vi "lifetime_error_buffer.vi"(1 "error in":errorcluster, 2 "command":string) -> (0 "error out":errorcluster)   [LabVIEW 2015]
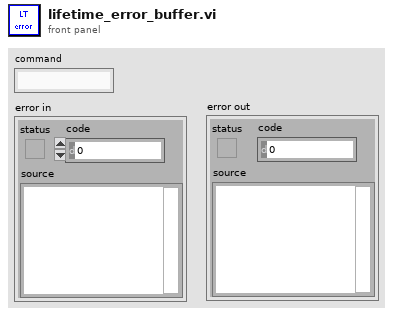
[diagram p1: front panel]
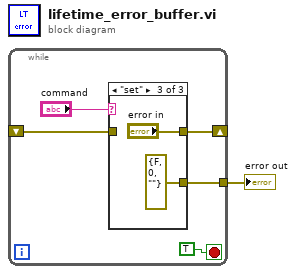
[diagram p0: block diagram]
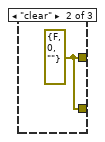
[diagram p3: hidden frame]
diagram:
  n1 = while {
    shift-right: [w4] -> _
    shift-left: _ -> [w3]
    tunnel: [w2] -> w1
    stop <- TRUE stop-if-true
    n2 = case shown="\"set\"" "command" {
      tunnel: [w7 w8 "error in"] -> w4
      tunnel: w3 -> [w7 _ _]
      tunnel: [w7 w8 errorcluster {"status"=FALSE, "code"=0, "source"=""} ("E_AI")] -> w2
      frame "get", Default {
      }
      frame "clear" {
        w8 = errorcluster {"status"=FALSE, "code"=0, "source"=""} ("E_AI")
      }
      frame "set" {
      }
    }
  }
  "error out" <- w1
